vi "FTW-TestExecutive-Start.vi"(0 "FTW Actor Connector In":refnum<class "FTW-ActorConnector.lvclass">, 11 "error in (no error)":errorcluster) -> (4 "FTW Actor Connector":refnum<class "FTW-ActorConnector.lvclass">, 14 "Roundtrip Time":dbl format="%.6f sec", 15 "error out":errorcluster)   [LabVIEW 2015]
uses:
  Connector/FTW-ActorConnector.lvclass
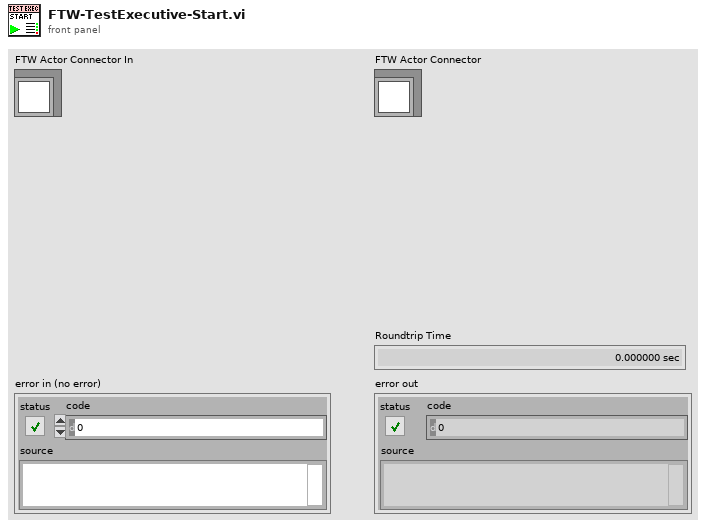
[diagram p1: front panel]
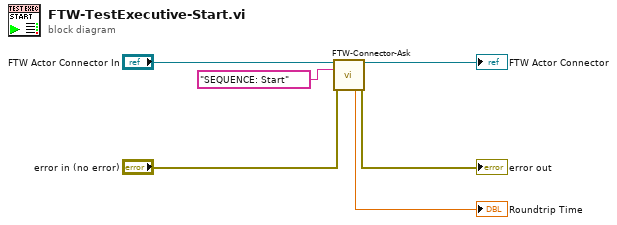
[diagram p0: block diagram]
diagram:
  n1 = call "FTW-Connector-Ask.vi"("FTW Actor Connector"="FTW Actor Connector In", "Request Header"="SEQUENCE: Start", "error in"="error in (no error)") -> ("FTW Actor Connector out"=→"FTW Actor Connector":refnum<class "FTW-ActorConnector.lvclass">, "Roundtrip Time"=→"Roundtrip Time":dbl, "error out"=→"error out":errorcluster)  [unwired: 7 in, 3 out]
